vi "UTILITY Get Column Stats.vi"(8 "Error In":errorcluster, 10 "Index":i32, 11 "Draw Stats":dbl[][](array[numeric])) -> (0 "Error Out":errorcluster, 3 "Column Stats":dbl[](array[numeric]))   [LabVIEW 2016]
uses:
  <vilib>/Analysis/NI_AALBase.lvlib
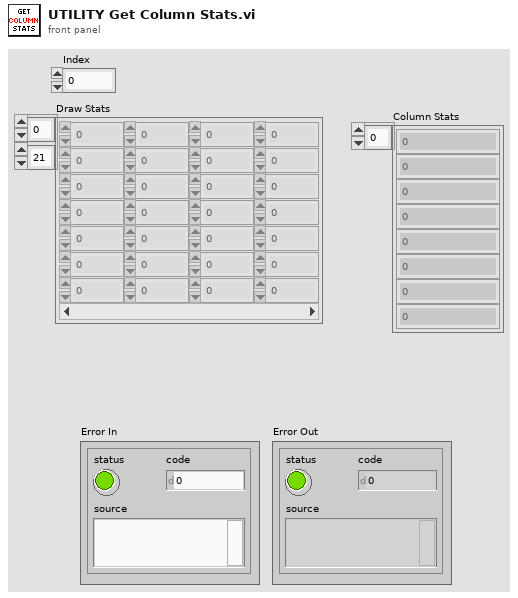
[diagram p1: front panel]
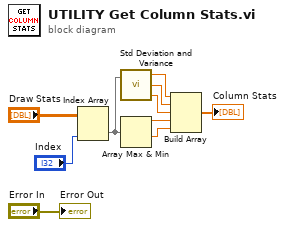
[diagram p0: block diagram]
diagram:
  n1 = Index Array(array="Draw Stats", index (col)="Index") -> (element=w4:dbl[])  [unwired: 1 in]
  n2 = call <vilib>:"Std Deviation and Variance.vi"("X"=w4) -> ("mean"=w5:dbl, "standard deviation"=w6:dbl, "variance"=w7:dbl)  [unwired: 1 in]
  n3 = Array Max & Min(array=w4) -> (max value=w8:dbl, min value=w9:dbl)  [unwired: 2 out]
  n4 = Build Array(w5, w6, w7, w8, w9) -> (→"Column Stats":dbl[])
  "Error Out" <- "Error In"
